vi "Write to Holding Register Channels.vi"(8 "error in (no error)":errorcluster, 9 "Holding Registers":T1[](array[typedef]) {"Mapping"."VS Reference" format="%.0x"}, 10 "Data In":dbl[](array[numeric]), 11 "Modbus Master in":refnum<class "Modbus Master.lvclass">=refnum) -> (0 "error out":errorcluster, 2 "Data Out":dbl[](array[numeric]), 3 "Modbus Master out":refnum<class "Modbus Master.lvclass">)   [LabVIEW 2021]
uses:
  Modbus API.lvlibp/API/Master/Modbus Master.lvclass
  System Explorer/SubVIs/Modbus Type.ctl
  Shared/Modbus Master Shared.lvlib
  Shared/Controls/Data Model/Channel.ctl
  Shared/Controls/Data Model/DataType.ctl
  Shared/Controls/Data Model/Mapping.ctl
  <vilib>/NI VeriStand/Custom Device API/Custom Device Channel Type.ctl
  <vilib>/NI VeriStand/Custom Device API/Custom Device API.lvlib
  <vilib>/NI VeriStand/Custom Device API/Custom Device Item Ref.ctl
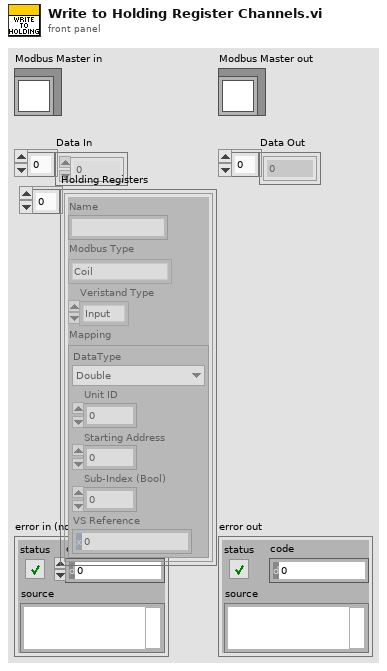
[diagram p1: front panel]
types:
  T1 = typedef "Modbus Master Shared.lvlib/Channel.ctl" = cluster{"Name":string, "Modbus Type":T2, "Veristand Type":T3, "Mapping":T4}
  T2 = typedef "Modbus Master Shared.lvlib/Modbus Type.ctl" = enum16{"Coil", "Discrete Input", "Holding Register", "Input Register"}
  T3 = typedef "Custom Device API.lvlib/Custom Device Channel Type.ctl" = enum16{"Input", "Output"}
  T4 = typedef "Modbus Master Shared.lvlib/Mapping.ctl" = cluster{"DataType":T5, "Unit ID":u8, "Starting Address":u16, "Sub-Index (Bool)":u16, "VS Reference":T6}
  T5 = typedef "Modbus Master Shared.lvlib/DataType.ctl" = enum16{"Double", "Single", "I64", "I32", "I16", "I8", "U64", "U32", "U16", "U8", "Boolean"}
  T6 = typedef "Custom Device API.lvlib/Custom Device Item Ref.ctl" = u64
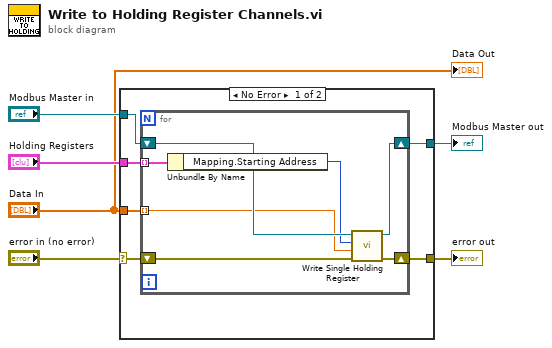
[diagram p0: block diagram]
diagram:
  n1 = case shown="No Error" "error in (no error)" {
    selector: "error in (no error)" -> [w12 w21]
    tunnel: [w11 w21] -> w5
    tunnel: "Holding Registers" -> [w10 _]
    tunnel: "Modbus Master in" -> [w9 w20]
    tunnel: [w8 w20] -> w2
    tunnel: "Data In" -> [w7 _]
    frame No Error {
      n2 = for {
        tunnel: w10 -> [w19] mode=indexing
        tunnel: w7 -> [w13] mode=indexing
        shift-right: [w18] -> w8
        shift-left: w9 -> [w17]
        shift-right: [w16] -> w11
        shift-left: w12 -> [w15]
        n3 = Unbundle By Name(w19) -> ("Mapping.Starting Address"=w14:u16)
        n4 = call-dynamic "Write Single Holding Register.vi"("error in"=w15, "register to write"=w13, "address"=w14, "Modbus master in"=w17) -> ("error out"=w16:errorcluster, "Modbus master out"=w18:refnum<class "Modbus Master.lvclass">)  [unwired: 6 in]
      }
    }
    frame Error {
    }
  }
  "error out" <- w5
  "Modbus Master out" <- w2
  "Data Out" <- "Data In"
